vi "ReadChnCfg.vi"(10 "num_chans":i32=16, 11 "Search Strings":string[](array[string])=["Verbose Name", "Units", "Sensitivity", "Offset"]) -> (2 "Table Minus Headers":string[][](array[string]), 3 "Full Table Output":string[][](array[string])=[["Verbose Name", "Units", "Sensitivity", "Offset", ""], ["P_2SPD_VENT", "bar a", "1", "", ""], ["P_OIL_2SPD_IN", "bar a", "2.05", "", ""], ["P_OIL_2SPD_SLND_OT", "bar a", "2.05", "", ""], ["P4_SPARE", "bar a", "", "", ""], ["P5_SPARE", "bar a", "", "", ""], ["P6_SPARE", "bar a", "", "", ""], ["P7_SPARE", "bar a", "", "", ""], ["P8_SPARE", "bar a", "", "", ""], ["RPM_2SPD_IN_FV", "rpm", "2362.2", "", ""], ["RPM_2SPD_OT_FV", "rpm", "2803.7", "", ""], ["T_2SPD_OIL_IN", "°C", "50", "", ""], ["T_2SPD_OIL_OT", "°C", "50", "", ""], ["TRQ_PMP_IN", "N·m", "20", "", ""], ["TRQ_2SPD_OT", "N·m", "10", "", ""], ["VFr_OIL_PTM_IN", "gpm", "7.25", "-7.25", ""], ["VFr_OIL_PUMP_OT", "gpm", "15", "-15", ""]])   [LabVIEW 2017]
uses:
  <vilib>/Utility/file.llb/Read Delimited Spreadsheet (string).vi
  <vilib>/regexp/Match Regular Expression.xnode
panel:
  out "Column":i32[](array[numeric])=[2, 10, 9, 11]
  out "Row":i32[](array[numeric])=[1, 1, 1, 1]
  out "all rows 2":string[](array[string])=["BNC Jack", "LabView Name", "Verbose Name", "Kistler SCP Assignment", "PXI Channel", "Range", "Voltage Divided?", "Sample Rate", "Sensor SN", "Sensitivity", "Units", "Offset", "Description", "", "", "", "", "\"v180406 updated channel name of \"\"HS_61\"\" to \"\"RPM_2SPD_OT_6602\"\"\"", "", "", "", "", "", "", "", "HS_40", "RPM_2SPD_OT_FV", "", ""]
  out "file or folder exists?":bool=TRUE
  out "all rows":string[][](array[string])=[["", "", "", "", "", "", "", "", "", "", "", "", "", "", "", "", "", "Revisions", "", "", "", "", "", "", "", "", "", "", ""], ["BNC Jack", "LabView Name", "Verbose Name", "Kistler SCP Assignment", "PXI Channel", "Range", "Voltage Divided?", "Sample Rate", "Sensor SN", "Sensitivity", "Units", "Offset", "Description", "", "", "", "", "\"v180406 updated channel name of \"\"HS_61\"\" to \"\"RPM_2SPD_OT_6602\"\"\"", "", "", "", "", "", "", "", "HS_40", "RPM_2SPD_OT_FV", "", ""], ["0", "P1", "P_2SPD_VENT", "", "\"Dev1, Ch 0\"", "", "No", "10 Hz", "DS1 SN20202", "1", "bar a", "", "Kistler  0-5 bar_a", "", "", "", "", "v181025 using channel map to build LabView waveforms for Orthrus oil pump performance testing", "", "", "", "", "", "", "", "HS_41", "P_2SPD_VENT", "", ""], ["1", "P2", "P_OIL_2SPD_IN", "", "\"Dev1, Ch 1\"", "", "No", "10 Hz", "", "2.05", "bar a", "", "Kistler  0-10 bar_a", "", "", "", "", "", "", "", "", "", "", "", "", "HS_42", "P_OIL_2SPD_IN", "", ""], ["2", "P3", "P_OIL_2SPD_SLND_OT", "", "\"Dev1, Ch 2\"", "", "Yes", "10 Hz", "", "2.05", "bar a", "", "Kistler  0-10 bar_a", "", "", "", "", "", "", "", "", "", "", "", "", "HS_43", "P_OIL_2SPD_SLND_OT", "", ""], ["3", "P4", "P4_SPARE", "", "\"Dev1, Ch 3\"", "", "Yes", "10 Hz", "", "", "bar a", "", "Kistler  0-10 bar_a", "", "", "", "", "", "", "", "", "", "", "", "", "HS_44", "T_2SPD_OIL_IN", "", ""], ["4", "P5", "P5_SPARE", "", "\"Dev1, Ch 4\"", "", "No", "10 Hz", "", "", "bar a", "", "Kistler  0-10 bar_a", "", "", "", "", "", "", "", "", "", "", "", "", "HS_45", "VFr_OIL_2SPD_IN", "", ""], ["5", "P6", "P6_SPARE", "", "\"Dev1, Ch 5\"", "", "No", "10 Hz", "", "", "bar a", "", "Kistler  0-10 bar_a", "", "", "", "", "", "", "", "", "", "", "", "", "HS_46", "TRQ_2SPD_DRVLN_OT", "", ""], ["6", "P7", "P7_SPARE", "", "\"Dev1, Ch 6\"", "", "No", "10 Hz", "", "", "bar a", "", "Kistler  0-10 bar_a", "", "", "", "", "", "", "", "", "", "", "", "", "HS_47", "RPM_2SPD_IN_FV", "", ""], ["7", "P8", "P8_SPARE", "", "\"Dev1, Ch 7\"", "", "No", "10 Hz", "", "", "bar a", "", "Kistler  0-10 bar_a", "", "", "", "", "", "", "", "", "", "", "", "", "HS_10", "TRQ_2SPD_OT", "", ""], ["8", "RPM_2SPD_IN_FV", "RPM_2SPD_IN_FV", "", "\"Dev2, Ch 0\"", "", "No", "10 Hz", "", "2362.2", "rpm", "", "\"Micro-epsilon turbo speed sensor reading 127PPR,  0-25kHz SCM5B45\"", "", "", "", "", "", "", "", "", "", "", "", "", "HS_11", "T_2SPD_OIL_OT", "", ""], ["9", "RPM_2SPD_OT_FV", "RPM_2SPD_OT_FV", "", "\"Dev2, Ch 1\"", "", "No", "10 Hz", "", "2803.7", "rpm", "", "\"Micro-epsilon turbo speed sensor reading 107 PPR, 0-25kHz SCM5B45\"", "", "", "", "", "", "", "", "", "", "", "", "", "HS_12", "HS_SPARE_12", "", ""], ["10", "T1", "T_2SPD_OIL_IN", "", "\"Dev2, Ch 2\"", "", "No", "10 Hz", "", "50", "°C", "", "Omega TXDIN70 Chn1", "", "", "", "", "", "", "", "", "", "", "", "", "HS_13", "TRQ_T22_2SPD_INPUT_PULLEY", "", ""], ["11", "T2", "T_2SPD_OIL_OT", "", "\"Dev2, Ch 3\"", "", "No", "10 Hz", "", "50", "°C", "", "Omega TXDIN70 Chn2", "", "", "", "", "", "", "", "", "", "", "", "", "HS_14", "HS_SPARE_14", "", ""], ["12", "TRQ1", "TRQ_PMP_IN", "", "\"Dev2, Ch 4\"", "", "No", "10 Hz", "", "20", "N·m", "", "Interface T22", "", "", "", "", "", "", "", "", "", "", "", "", "HS_15", "HS_SPARE_15", "", ""], ["13", "TRQ2", "TRQ_2SPD_OT", "", "\"Dev2, Ch 5\"", "", "Yes", "10 Hz", "", "10", "N·m", "", "HBM T21WN on 2SPD output shaft", "", "", "", "", "", "", "", "", "", "", "", "", "HS_16", "HS_SPARE_16", "", ""], ["14", "F1", "VFr_OIL_PTM_IN", "", "\"Dev2, Ch 6\"", "", "No", "10 Hz", "", "7.25", "gpm", "-7.25", "0-29 gpm Hoffer flowmeter", "", "", "", "", "", "", "", "", "", "", "", "", "HS_17", "HS_SPARE_17", "", ""], ["15", "F2", "VFr_OIL_PUMP_OT", "", "\"Dev2, Ch 7\"", "", "No", "10 Hz", "", "15", "gpm", "-15", "0-60 gpm Hoffer flowmeter", "", "", "", "", "", "", "", "", "", "", "", "", "HS_60", "RPM_DRVLN_6602", "", ""], ["PFI38", "RPM_DRVLN_6602", "RPM_DRVLN_6602", "", "\"Dev3, Ctr 0\"", "", "No", "80MHz Timebase", "", "", "", "", "Driveline speed measure without any multipliers.  Minimum pulse width filter set to 1E-5 s.", "", "", "", "", "", "", "", "", "", "", "", "", "HS_61", "RPM_2SPD_OT_6602", "", ""], ["PFI23", "RPM_2SPD_OT_6602", "RPM_2SPD_OT_6602", "", "\"Dev3, Ctr 1\"", "", "No", "80MHz Timebase", "", "", "", "", "2Spd Drive output speed.  Minimum pulse width filter set to 1E-5 s.", "", "", "", "", "", "", "", "", "", "", "", "", "HS_62", "", "", ""], ["", "", "HS_62", "", "\"Dev3, Ctr 2\"", "", "No", "80MHz Timebase", "", "", "", "", "", "", "", "", "", "", "", "", "", "", "", "", "", "HS_63", "", "", ""], ["", "", "HS_63", "", "\"Dev3, Ctr 3\"", "", "No", "80MHz Timebase", "", "", "", "", "", "", "", "", "", " ", "", "", "", "", "", "", "", "HS_64", "", "", ""], ["", "", "HS_64", "", "\"Dev3, Ctr 4\"", "", "No", "80MHz Timebase", "", "", "", "", "", "", "", "", "", "", "", "", "", "", "", "", "", "HS_65", "", "", ""], ["", "", "HS_65", "", "\"Dev3, Ctr 5\"", "", "No", "80MHz Timebase", "", "", "", "", "", "", "", "", "", "", "", "", "", "", "", "", "", "HS_66", "", "", ""], ["", "", "HS_66", "", "\"Dev3, Ctr 6\"", "", "No", "80MHz Timebase", "", "", "", "", "", "", "", "", "", "", "", "", "", "", "", "", "", "HS_67", "", "", ""], ["", "", "HS_67", "", "\"Dev3, Ctr 7\"", "", "No", "80MHz Timebase", "", "", "", "", "", "", "", "", "", "", "", "", "", "", "", "", "", "", "", "", ""], ["", "", "", "", "", "", "", "", "", "", "", "", "", "", "", "", "", "", "", "", "", "", "", "", "", "2362.204724", "", "5000", "Hz/Volt"], [" ", "", "", "", "", "", "", "", "", "", "", "", "", "", "", "", "", "", "", "", "", "", "", "", "", "24", "rev/block", "127", "Hz/rev @ 1 rps"], ["", "", "", "", "", "", "", "", "", "", "", "", "", "", "", "", "", "", "", "", "", "", "", "", "", "", "", "39.37007874", "rev/Volt-s"], ["", "", "", "", "", "", "", "", "", "", "", "", "", "", "", "", "", "", "", "", "", "", "", "", "", "", "", "2362.204724", "rev/Volt-minute"], ["", "", "", "1015", "", "", "", "", "", "", "", "", "", "", "", "", "", "", "", "", "", "", "", "", "", "", "", "", ""], ["", "", "", "", "", "", "", "", "", "", "", "", "", "", "", "", "", "", "", "", "", "", "", "", "", "", "", "", ""], ["", "", "", "", "", "", "", "", "", "", "", "", "", "", "", "", "", "", "", "", "", "", "", "", "", "", "2.538", "Pulley ratio", ""], ["", "", "", "", "", "", "", "", "", "", "", "", "", "", "", "", "", "", "", "", "", "", "", "", "", "", "1.186915888", "2Spd Drive Ratio", ""], ["", "", "", "", "", "", "", "", "", "", "", "", "", "", "", "", "", "", "", "", "", "", "", "", "", "", "1050", "RPM Motor", ""], ["", "", "", "", "", "", "", "", "", "", "", "", "", "", "", "", "", "", "", "", "", "", "", "", "", "", "", "", ""], ["", "", "", "", "", "", "", "", "", "", "", "", "", "", "", "", "", "", "", "", "", "", "", "", "", "", "3163.01215", "RPM_2SPD_OT", ""], ["", "", "", "", "", "", "", "", "", "", "", "", "", "", "", "", "", "", "", "", "", "", "", "", "", "", "8640", "360", ""]]
  # "This VI searches a \"spreadsheed.txt\" tab-delimted file (e.g. exported from Excel) for column headers that contain certain strings.  It then grabs the column\nassociated with that header and \"num_channels\" of rows below each header.\nv190610_A updated to point to current VI directory & \"\\ChnCfg.txt\" for channels file."
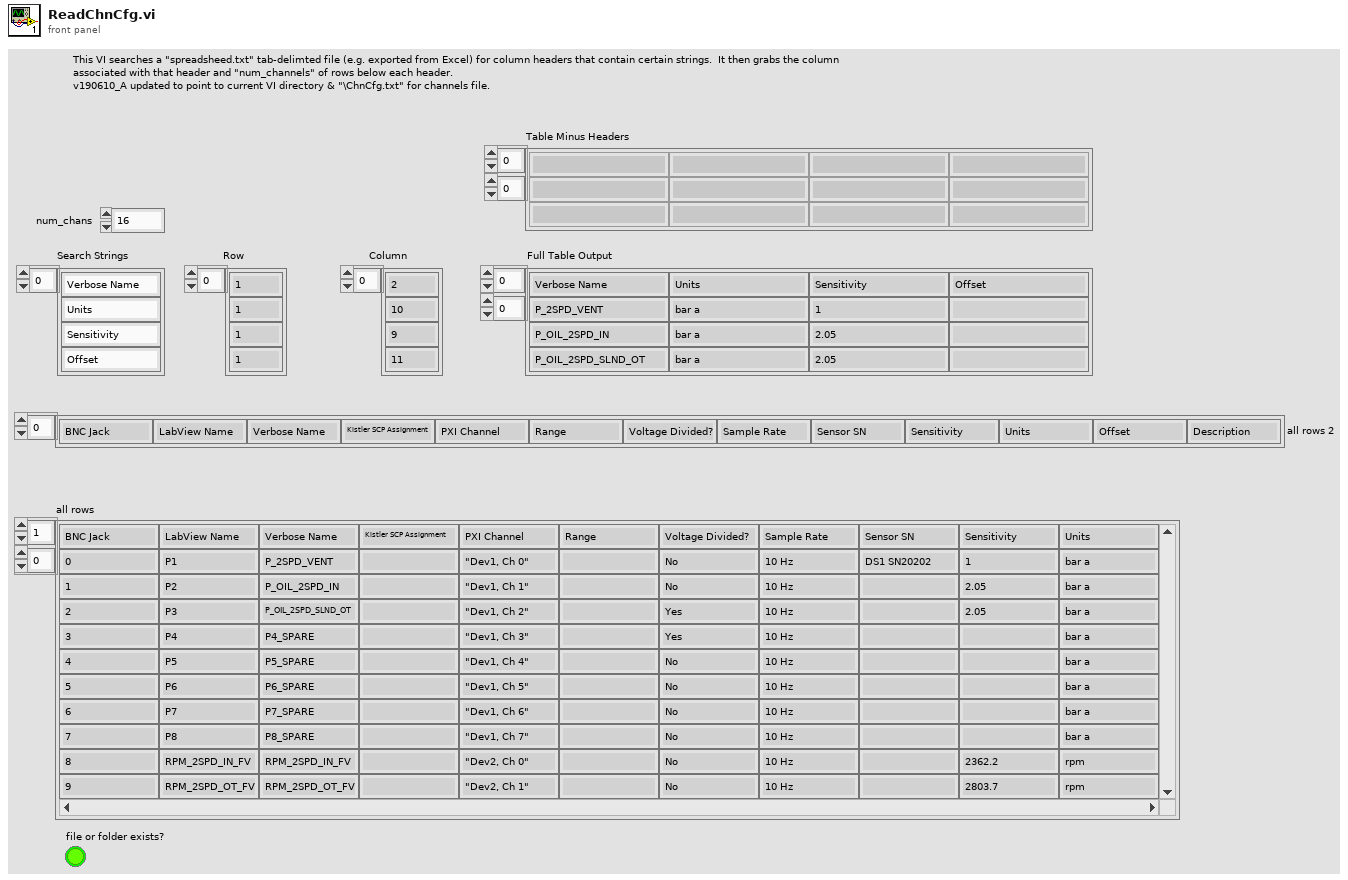
[diagram p1: front panel]
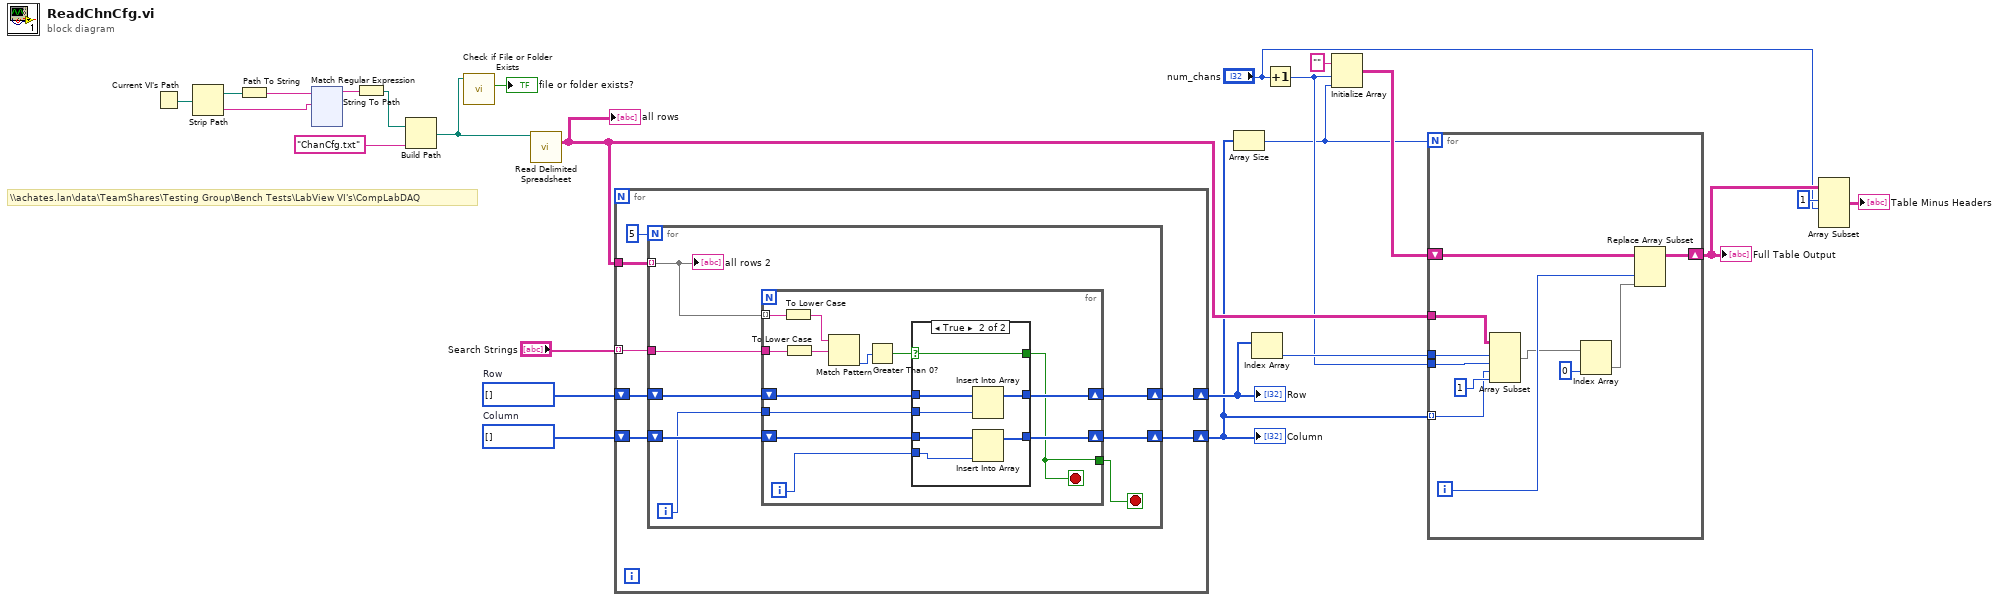
[diagram p0: block diagram]
diagram:
  w21 = i32[] []  # Column
  w22 = i32[] []  # Row
  # "\\\\achates.lan\\data\\TeamShares\\Testing Group\\Bench Tests\\LabView VI's\\CompLabDAQ"
  n1 = Current VI's Path() -> (path=w6:path)
  n2 = Strip Path(path=w6) -> (stripped path=w5:path, name=w3:string)
  n3 = Path To String(path=w5) -> (string=w4:string)
  n4 = xnode "Match Regular Expression"("input string"=w4, "regular expression"=w3) -> ("before match"=w2:string)  [unwired: 4 in, 4 out]
  n5 = String To Path(string=w2) -> (path=w1:path)
  n6 = Build Path(base path=w1, name or relative path="ChanCfg.txt") -> (appended path=w7:path)
  n7 = call <vilib>:"Check if File or Folder Exists.vi"("path"=w7) -> ("file or folder exists?"=→"file or folder exists?":bool)  [unwired: 8 in, 2 out]
  n8 = call-poly <vilib>:"Read Delimited Spreadsheet.vi"("file path (dialog if empty)"=w7) -> ("all rows"=w20:string[][])  [unwired: 9 in, 5 out]
  "all rows" <- w20
  n9 = for {
    tunnel: "Search Strings" -> [w30] mode=indexing
    tunnel: w20 -> [w27]
    shift-right: [w26] -> w19
    shift-left: w22 -> [w29]
    shift-right: [w25] -> w15
    shift-left: w21 -> [w28]
    n10 = for {
      N: 5 -> [_]
      tunnel: w27 -> [w39] mode=indexing
      tunnel: w30 -> [w38]
      shift-right: [w34] -> w26
      shift-left: w29 -> [w37]
      shift-right: [w33] -> w25
      shift-left: w28 -> [w36]
      i -> [w35]
      stop <- w32 stop-if-true
      n11 = for {
        tunnel: w39 -> [w50] mode=indexing
        tunnel: w38 -> [w49]
        tunnel: w35 -> [w44]
        shift-right: [w42] -> w34
        shift-left: w37 -> [w46]
        shift-right: [w41] -> w33
        shift-left: w36 -> [w45]
        tunnel: [w40] -> w32
        i -> [w43]
        stop <- w40 stop-if-true
        n12 = To Lower Case(string=w50) -> (all lower case string=w52:string)
        n13 = To Lower Case(string=w49) -> (all lower case string=w51:string)
        n14 = Match Pattern(string=w52, regular expression=w51) -> (offset past match=w48:i32)  [unwired: 1 in, 3 out]
        n15 = Greater Than 0?(x=w48) -> (x > 0?=w47:bool)
        n16 = case shown="True" w47 {
          selector: w47 -> [w53 w56]
          tunnel: w46 -> [w55 w62]
          tunnel: w45 -> [w54 w60]
          tunnel: w44 -> [_ w61]
          tunnel: w43 -> [_ w59]
          tunnel: [w55 w58] -> w42
          tunnel: [w54 w57] -> w41
          tunnel: [w53 w56] -> w40
          frame False {
          }
          frame True {
            n17 = Insert Into Array(array=w62, new element=w61) -> (w58:i32[])  [unwired: 1 in]
            n18 = Insert Into Array(array=w60, new element=w59) -> (w57:i32[])  [unwired: 1 in]
          }
        }
      }
      "all rows 2" <- w39
    }
  }
  "Row" <- w19
  "Column" <- w15
  n19 = Array Size(array=w15) -> (size(s)=w9:i32)
  n20 = Index Array(array=w19) -> (element=w18:i32)  [unwired: 1 in]
  n21 = Increment(x="num_chans") -> (x+1=w14:i32)
  n22 = Initialize Array("", w14, w9) -> (w16:string[][])
  n23 = for {
    N: w9 -> [_]
    tunnel: w20 -> [w72]
    tunnel: w18 -> [w71]
    shift-right: [w66] -> w13
    shift-left: w16 -> [w73]
    tunnel: w15 -> [w65] mode=indexing
    tunnel: w14 -> [w63]
    i -> [w69]
    n24 = Array Subset(array=w72, index (row)=w71, length (row)=w63, index (col)=w65, length (col)=1 ("length")) -> (w68:string[][])
    n25 = Index Array(array=w68, index (col)=0 ("disabled index (col)")) -> (element=w67:string[])  [unwired: 1 in]
    n26 = Replace Array Subset(array=w73, new element=w67, index (col)=w69) -> (w66:string[][])  [unwired: 1 in]
  }
  "Full Table Output" <- w13
  n27 = Array Subset(array=w13, index (row)=1 ("index"), length (row)="num_chans") -> (→"Table Minus Headers":string[][])  [unwired: 2 in]
